vi "Deconstruct.vi"(0 "Component in":refnum<class "Component.lvclass">) -> ()   [LabVIEW 2017, in "CL_G3_VIComponentBuilder.lvlib" / "Component.lvclass"]
doc: "Destroys the Component object."
uses:
  Component.lvclass
  Exports/Exports/Export.lvclass
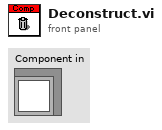
[diagram p1: front panel]
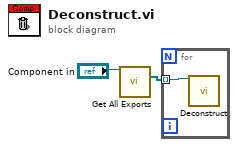
[diagram p0: block diagram]
diagram:
  n1 = call "Get All Exports.vi"("Component in"="Component in") -> ("Exports"=w1:refnum<class "Export.lvclass">[])  [unwired: 13 in, 1 out]
  n2 = for {
    tunnel: w1 -> [w3] mode=indexing
    n3 = call-dynamic "Deconstruct.vi"("Export In"=w3) -> ()  [unwired: 15 in]
  }
